vi "nPoints Concept - Potentiometer.vi"() -> ()   [LabVIEW 2014]
panel:
  out "Acquired Voltage":dbl min=0.0 max=100.0 step=1.0 format="%.2f"
  out "Linear Potentiometer":dbl(slide) scale=0.0..5.0
  out "Radial Potentiometer":dbl(knob) scale=0.0..5.0
  in  "Stop Button":bool
  # "Potentiometer"
  # "5V"
  # "GND"
  # "CCW\n(GND)"
  # "CW\n(5V)"
  # "Signal"
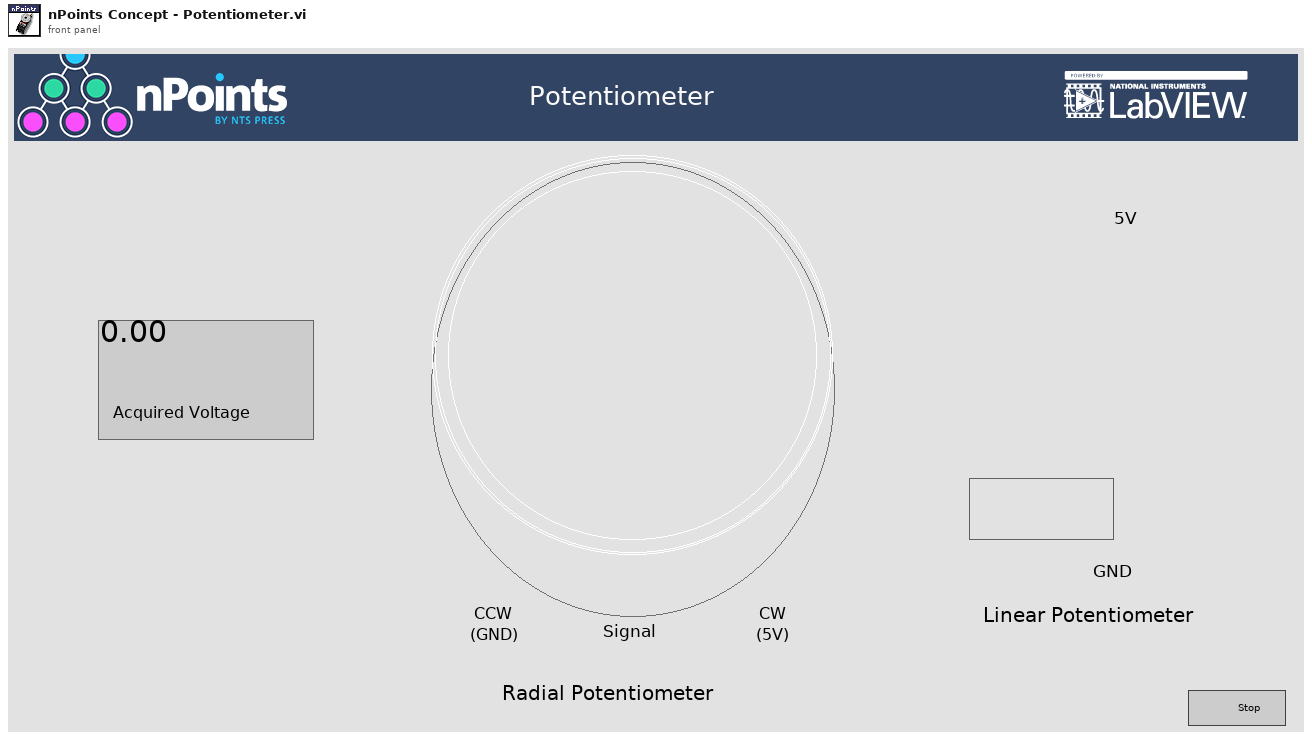
[diagram p1: front panel]
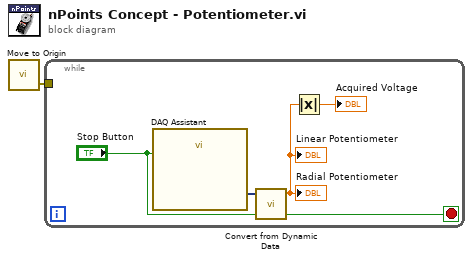
[diagram p0: block diagram]
diagram:
  n1 = call <userlib>:"Move to Origin.vi"() -> ("Error Out"=w1:errorcluster)  [unwired: 3 in]
  n2 = while {
    tunnel: w1 -> [_]
    stop <- "Stop Button" stop-if-true
    n3 = call "DAQ Assistant"("stop (T)"="Stop Button") -> ("data"=w5:dynamicdata)  [unwired: 16 in, 2 out]
    n4 = call "Convert from Dynamic Data"("Dynamic Data Type"=w5) -> ("Scalar"=w3:dbl)  [unwired: 3 in]
    "Radial Potentiometer" <- w3
    "Linear Potentiometer" <- w3
    n5 = Absolute Value(x=w3) -> (abs(x)=→"Acquired Voltage":dbl)
  }
